vi "Obciecie zer.vi"(11 "Wejściowa liczba":string) -> (3 "Wyjściowa liczba":string)   [LabVIEW 2020]
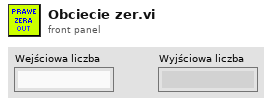
[diagram p1: front panel]
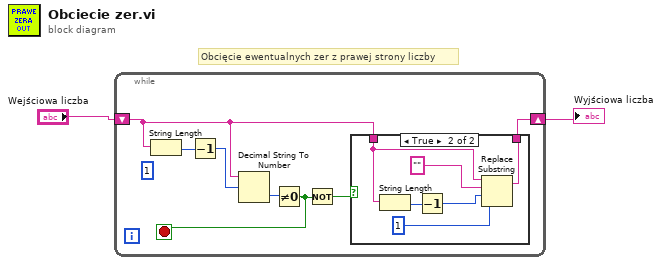
[diagram p0: block diagram]
diagram:
  # "Obcięcie ewentualnych zer z prawej strony liczby"
  n1 = while {
    shift-right: [w4] -> w1
    shift-left: "Wejściowa liczba" -> [w3]
    stop <- w6 stop-if-true
    (unwired) 1 ("length (len. of substring)")
    n2 = String Length(string=w3) -> (length=w8:i32)
    n3 = Decrement(x=w8) -> (x-1=w7:i32)
    n4 = Decimal String To Number(string=w3, offset=w7) -> (number=w9:i32)  [unwired: 1 in, 1 out]
    n5 = Not Equal To 0?(x=w9) -> (x != 0?=w6:bool)
    n6 = Not(x=w6) -> (.not. x?=w5:bool)
    n7 = case shown="True" w5 {
      tunnel: [w10 w12] -> w4
      tunnel: w3 -> [w10 w11]
      frame False {
      }
      frame True {
        n8 = String Length(string=w11) -> (length=w15:i32)
        n9 = Decrement(x=w15) -> (x-1=w14:i32)
        n10 = Replace Substring(2:1 ("length (len. of substring)"), 3:w14, 4:"" ("substring (\"\")"), 5:w11) -> (1:w12:string)  [unwired: 1 out]
      }
    }
  }
  "Wyjściowa liczba" <- w1
